vi "FTP_VIEWER.vi"() -> ()   [LabVIEW 2026]
uses:
  <vilib>/FTP/ftp2.llb/FTP File Info.ctl
  <vilib>/FTP/NI_FTP.lvlib
panel:
  out "dir list[0].name":string
  out "reply string 2":string
  in  "directory path":string
  out "dir list":T1[](array[typedef])
  out "reply string":string
  out "reply code":i32
  out "reply out":string
  in  "password":string
  in  "user":string="anonymous"
  in  "timeout ms":i32=60000
  in  "remote port (21)":u16=21
  in  "address":string
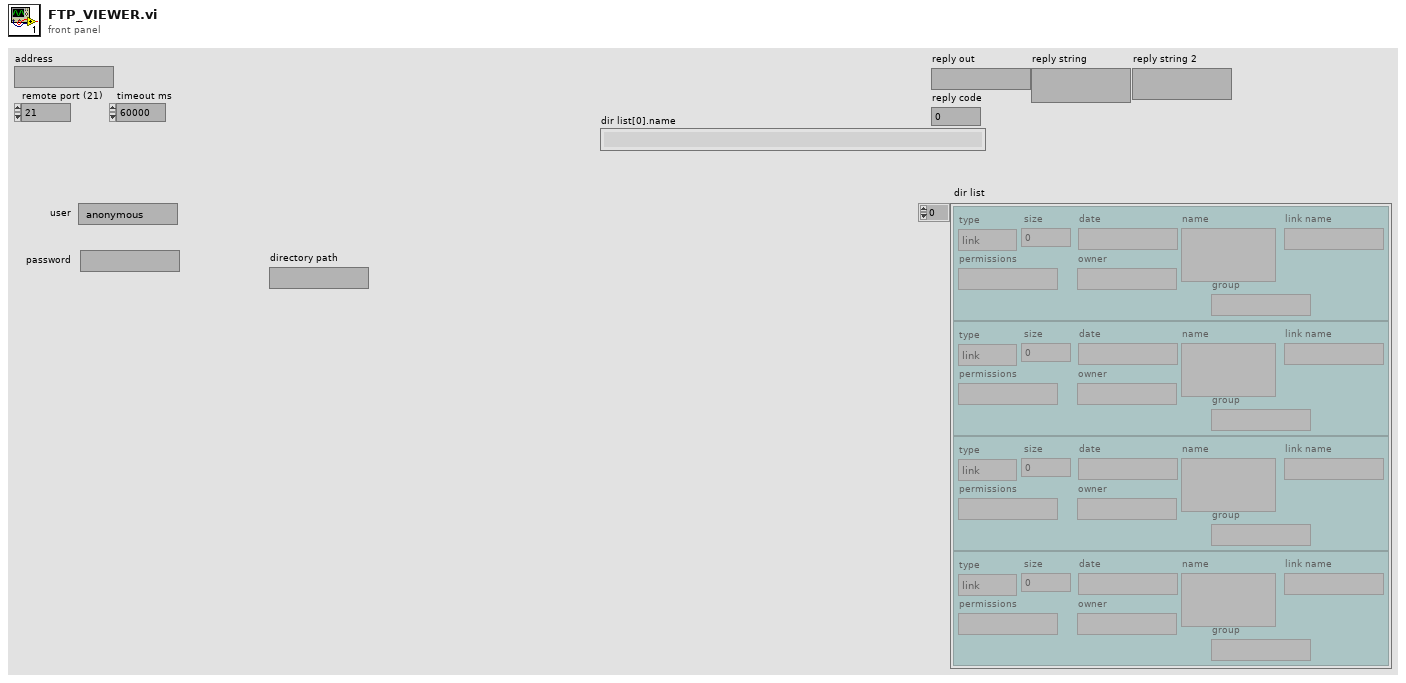
[diagram p1: front panel]
types:
  T1 = typedef "NI_FTP.lvlib/FTP File Info.ctl" = cluster{"type":enum16{"unknown", "file", "dir", "link"}, "permissions":string, "owner":string, "group":string, "size":i32, "date":string, "name":string, "link name":string}
  T2 = typedef "NI_FTP.lvlib/FTP Session.ctl" = refnum<k5>
  T3 = cluster{"dir list[0]":T1, "dir list[1]":T1, "dir list[2]":T1, "dir list[3]":T1, "dir list[4]":T1, "dir list[5]":T1, "dir list[6]":T1, "dir list[7]":T1, "dir list[8]":T1}
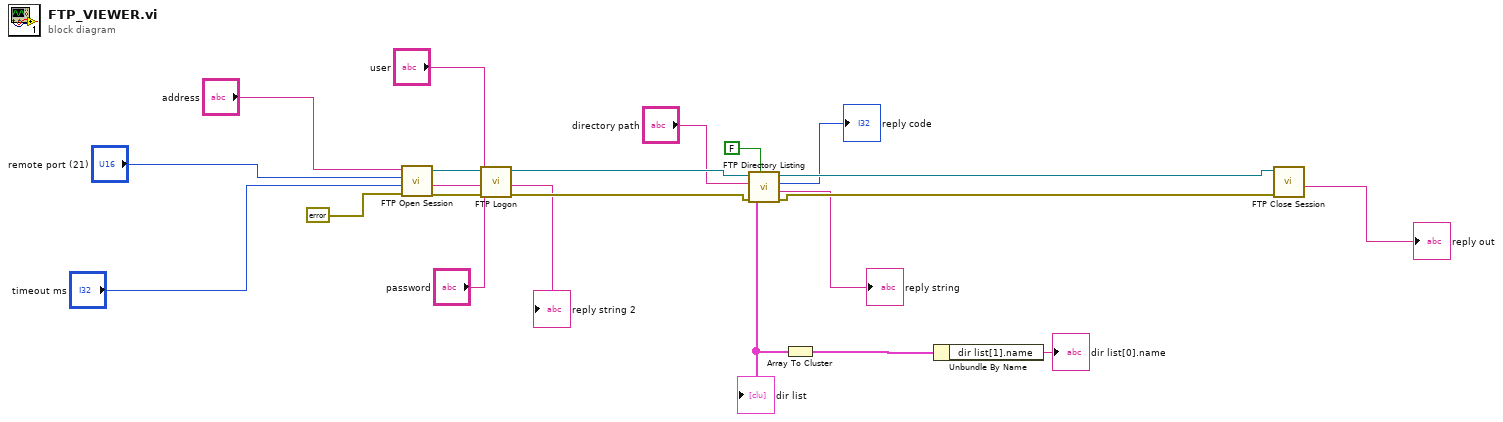
[diagram p0: block diagram]
diagram:
  n1 = call <vilib>:"FTP Open Session.vi"("error in (no error)"=errorcluster {"status"=FALSE, "code"=0, "source"=""}, "timeout ms (60000)"="timeout ms", "remote port (21)"="remote port (21)", "address"="address") -> ("error out"=w14:errorcluster, "reply string"=→"reply string 2":string, "ftp session"=w17:T2)  [unwired: 4 in, 1 out]
  n2 = call <vilib>:"FTP Logon.vi"("error in (no error)"=w14, "password"="password", "user"="user", "ftp session"=w17) -> ("error out"=w12:errorcluster, "ftp session out"=w13:T2)  [unwired: 4 in, 2 out]
  n3 = call <vilib>:"FTP Directory Listing.vi"("active (T)"=FALSE, "error in (no error)"=w12, "directory path"="directory path", "ftp session"=w13) -> ("error out"=w11:errorcluster, "reply string"=→"reply string":string, "reply code"=→"reply code":i32, "ftp session out"=w10:T2, "dir list"=w3:T1[])  [unwired: 3 in]
  "dir list" <- w3
  n4 = Array To Cluster(array=w3) -> (cluster=w2:T3)
  n5 = Unbundle By Name(w2) -> ("dir list[1].name"=→"dir list[0].name":string)
  n6 = call <vilib>:"FTP Close Session.vi"("error in (no error)"=w11, "ftp session"=w10) -> ("reply string"=→"reply out":string)  [unwired: 6 in, 3 out]
